vi "laba3.2.vi"() -> ()   [LabVIEW 2018]
panel:
  out "-":dbl[](array[numeric])
  out "+":dbl[](array[numeric])
  in  "вход":dbl[](array[numeric])
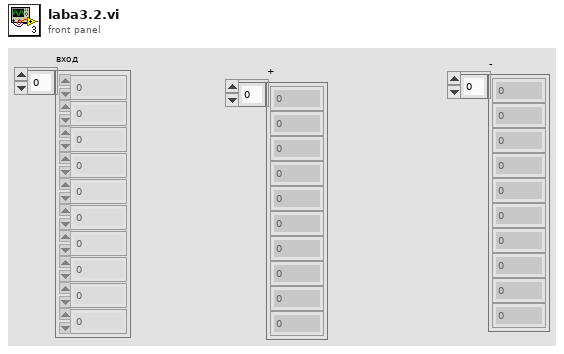
[diagram p1: front panel]
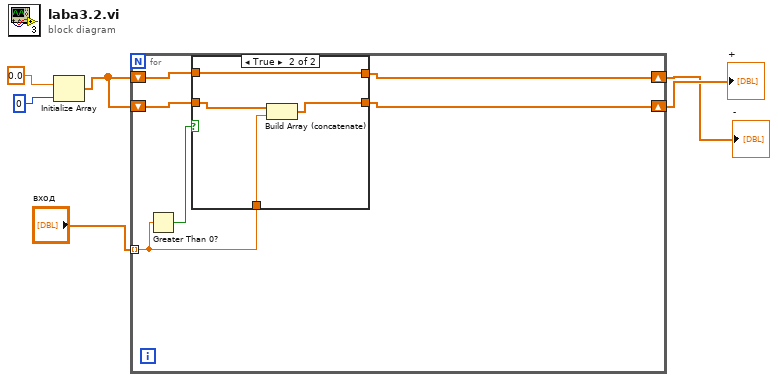
[diagram p0: block diagram]
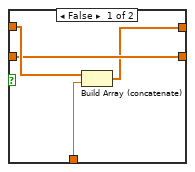
[diagram p2: hidden frame]
diagram:
  n1 = Initialize Array(0.0, 0) -> (w3:dbl[])
  n2 = for {
    shift-right: [w8] -> w1
    shift-left: w3 -> [w12]
    shift-right: [w7] -> w2
    shift-left: w3 -> [w10]
    tunnel: "вход" -> [w9] mode=indexing
    n3 = Greater Than 0?(x=w9) -> (x > 0?=w11:bool)
    n4 = case shown="True" w11 {
      tunnel: w12 -> [w16 w20]
      tunnel: w10 -> [w14 w19]
      tunnel: w9 -> [w15 w18]
      tunnel: [w14 w17] -> w7
      tunnel: [w13 w20] -> w8
      frame False {
        n5 = Build Array (concatenate)(w16, w15) -> (w13:dbl[])
      }
      frame True {
        n6 = Build Array (concatenate)(w19, w18) -> (w17:dbl[])
      }
    }
  }
  "+" <- w2
  "-" <- w1
